vi "Get_Default_Dest.vi"(8 "error in (no error)":errorcluster, 11 "Installer in":refnum<class "Installer.lvclass">) -> (0 "error out":errorcluster, 2 "found?":bool, 3 "IB_Destination.lvclass":refnum<class "IB_Destination.lvclass">)   [LabVIEW 2020, in "Installer.lvclass"]
uses:
  <vilib>/AppBuilder/IB_Classes/Installer/Installer.lvclass
  <vilib>/AppBuilder/IB_Classes/Installer/Installer.lvclass/Installer.ctl
  <vilib>/AppBuilder/IB_Classes/Destination/IB_Destination.lvclass
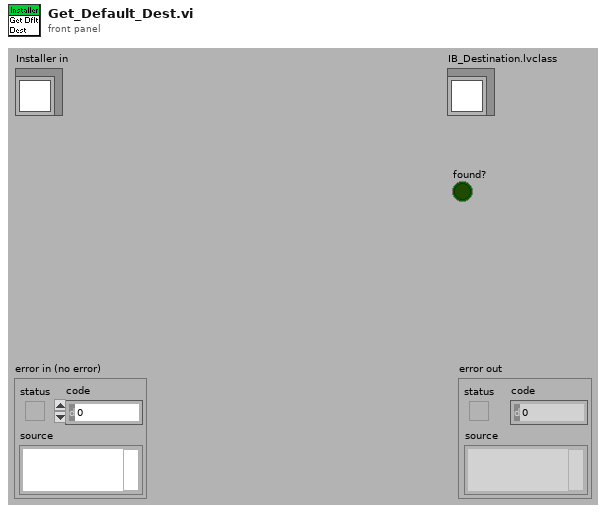
[diagram p1: front panel]
types:
  T1 = typedef "IB_Destination.ctl" = cluster{"name":string, "unlock":bool, "parentTag":string, "destTag":string, "eng_installPath":string}
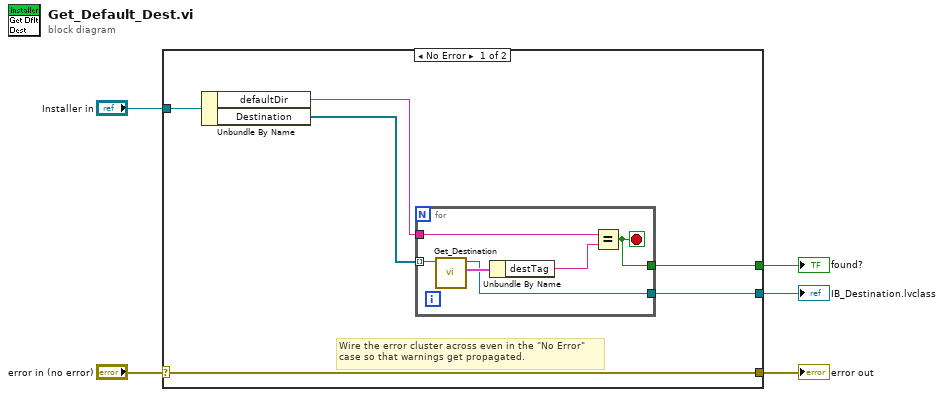
[diagram p0: block diagram]
diagram:
  n1 = case shown="No Error" "error in (no error)" {
    selector: "error in (no error)" -> [w11 w18]
    tunnel: [w11 w18] -> w4
    tunnel: "Installer in" -> [w8 _]
    tunnel: [w7 _] -> w2
    tunnel: [w6 _] -> w1
    frame No Error {
      # "Wire the error cluster across even in the \"No Error\"\ncase so that warnings get propagated."
      n2 = Unbundle By Name(w8) -> ("defaultDir"=w9:string, "Destination"=w10:refnum<class "IB_Destination.lvclass">[])
      n3 = for {
        tunnel: w10 -> [w17] mode=indexing
        tunnel: w9 -> [w15]
        tunnel: [w13] -> w7
        tunnel: [w12] -> w6
        stop <- w12 stop-if-true
        n4 = call <vilib>:"Get_Destination.vi"("IB_Destination in"=w17) -> ("data"=w16:T1, "IB_Destination out"=w13:refnum<class "IB_Destination.lvclass">)  [unwired: 1 in, 8 out]
        n5 = Unbundle By Name(w16) -> ("destTag"=w14:string)
        n6 = Equal?(x=w15, y=w14) -> (x = y?=w12:bool)
      }
    }
    frame Error {
    }
  }
  "error out" <- w4
  "IB_Destination.lvclass" <- w2
  "found?" <- w1
